vi "Motor controller.vi"   [LabVIEW 2012]
uses:
  Motors Values.vi
  BotStatus.vi
types:
  T1 = typedef "WPI_ServoDeviceRef.ctl" = cluster{"DeviceStatus":errorcluster, "Digital Module":T2, "PWM Channel":T3, "DeadBand":T4}
  T2 = typedef "FPGA_TypedefDigitalModule.ctl" = enum16{"Digital Module 1", "Digital Module 2"}
  T3 = typedef "FPGA_DIOPWMChannel.ctl" = enum8{"PWM 1", "PWM 2", "PWM 3", "PWM 4", "PWM 5", "PWM 6", "PWM 7", "PWM 8", "PWM 9", "PWM 10", "Invalid"}
  T4 = typedef "WPI_PWMDeadband.ctl" = cluster{"Name":string, "maxPositivePwm":i32, "minPositivePwm":i32, "centerPwm":i32, "maxNegativePwm":i32, "minNegativePwm":i32, "angularRange":u16}
  T5 = typedef "WPI_MotorControlDeviceRef.ctl" = cluster{"DeviceStatus":errorcluster, "Type":enum16{"PWM", "CAN"}, "PWM":cluster{"Digital Module":T2, "PWM Channel":T3, "DeadBand":T4}, "CAN":cluster{"Device Number":u8, "Control Mode":T6, "Semaphore":T7, "Max Vout":dbl}, "Invert":bool, "TransformRef":T8, "InvTransformRef":T8}
  T6 = typedef "WPI_CANJaguar_ControlMode.ctl" = enum8{"Percent VBus", "Current", "Speed", "Position", "Voltage"}
  T7 = typedef "Semaphore RefNum" = refnum<k1>
  T8 = typedef "WPI_PWMTransform_ConPane.ctl" = refnum<vi>
  T9 = typedef "WPI_RelayDevRef.ctl" = cluster{"DevStatus":errorcluster, "Relay Channel":T10, "Digital Module":T2, "Relay Direction":T11}
  T10 = typedef "FPGA_DIORelayChannel.ctl" = enum8{"Relay 1", "Relay 2", "Relay 3", "Relay 4", "Relay 5", "Relay 6", "Relay 7", "Relay 8", "Invalid"}
  T11 = typedef "WPI_RelayDirection.ctl" = enum16{"Both directions", "Forward only", "Reverse only"}
  T12 = typedef "WPI_RelayValue.ctl" = enum16{"Off", "On", "Forward", "Reverse"}
  T13 = typedef "WPI_DigitalInputDevRef.ctl" = cluster{"DevStatus":errorcluster, "DIO Channel":T14, "Digital Module":T2}
  T14 = typedef "FPGA_DIOChannel.ctl" = enum8{"DIO 1", "DIO 2", "DIO 3", "DIO 4", "DIO 5", "DIO 6", "DIO 7", "DIO 8", "DIO 9", "DIO 10", "DIO 11", "DIO 12", "DIO 13", "DIO 14", "Invalid"}
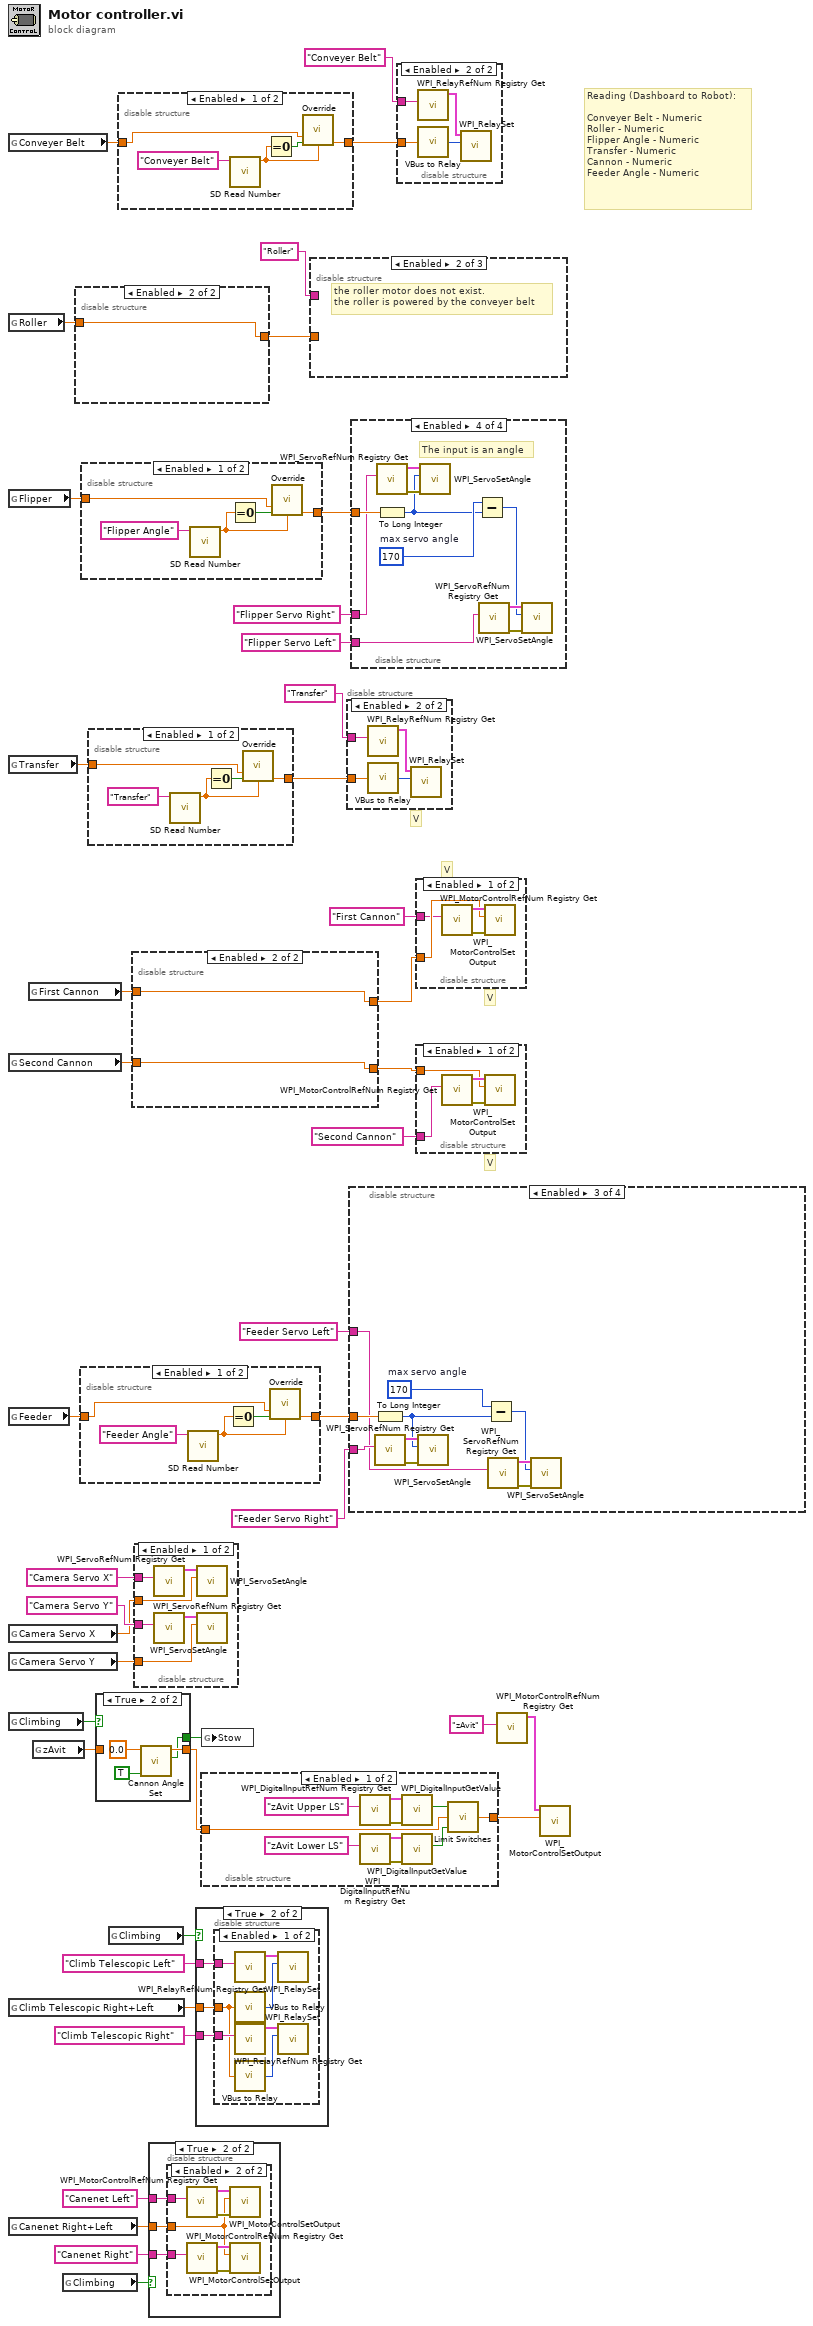
[diagram p0: block diagram]
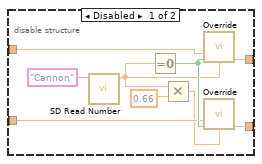
[diagram p4: hidden frame]
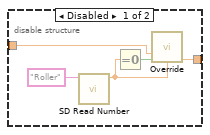
[diagram p7: hidden frame]
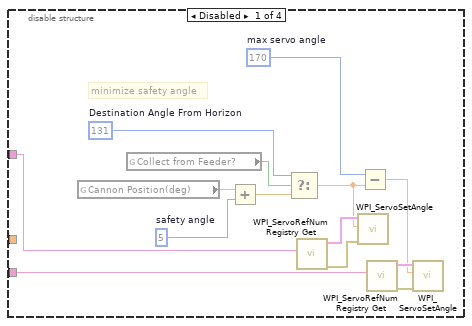
[diagram p10: hidden frame]
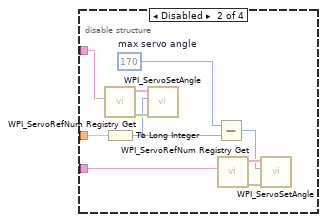
[diagram p11: hidden frame]
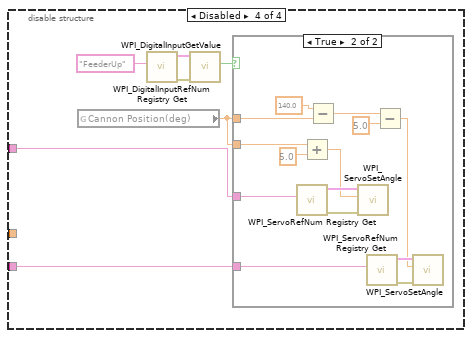
[diagram p12: hidden frame]
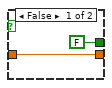
[diagram p14: hidden frame]
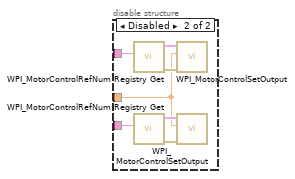
[diagram p18: hidden frame]
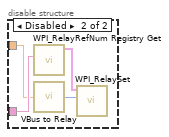
[diagram p19: hidden frame]
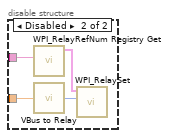
[diagram p20: hidden frame]
diagram:
  # "Reading (Dashboard to Robot):\n\nConveyer Belt - Numeric\nRoller - Numeric\nFlipper Angle - Numeric\nTransfer - Numeric\nCannon - Numeric\nFeeder Angle - Numeric"
  # "V"
  # "V"
  # "V"
  # "V"
  n1 = global read "Motors Values.vi" "Conveyer Belt"() -> (w15:dbl)
  n2 = global read "Motors Values.vi" "Roller"() -> (w14:dbl)
  n3 = global read "Motors Values.vi" "Flipper"() -> (w12:dbl)
  n4 = global read "Motors Values.vi" "Transfer"() -> (w10:dbl)
  n5 = global read "Motors Values.vi" "Second Cannon"() -> (w6:dbl)
  n6 = global read "Motors Values.vi" "Feeder"() -> (w3:dbl)
  n7 = global read "Motors Values.vi" "Camera Servo X"() -> (w18:dbl)
  n8 = global read "Motors Values.vi" "Camera Servo Y"() -> (w17:dbl)
  n9 = global read "BotStatus.vi" "Climbing"() -> (w26:bool)
  n10 = global read "Motors Values.vi" "Climb Telescopic Right+Left"() -> (w34:dbl)
  n11 = global read "Motors Values.vi" "Canenet Right+Left"() -> (w27:dbl)
  n12 = global read "Motors Values.vi" "First Cannon"() -> (w8:dbl)
  n13 = global read "Motors Values.vi" "zAvit"() -> (w25:dbl)
  n14 = global read "BotStatus.vi" "Climbing"() -> (w28:bool)
  n15 = disable-structure shown="Enabled" {
    disable-tunnel: w14 -> [w44 w48]
    disable-tunnel: [w43 w48] -> w13
    frame Disabled {
      n16 = call <vilib>:"SD Read Number.vi"("Name"="Roller") -> ("Numeric"=w46:dbl)  [unwired: 8 in, 2 out]
      n17 = Equal To 0?(x=w46) -> (x = 0?=w47:bool)
      n18 = call "Override.vi"("Regualer"=w44, "Override"=w47, "Overriden"=w46) -> ("Output"=w43:dbl)  [unwired: 12 in]
    }
    frame Enabled {
    }
  }
  n19 = disable-structure shown="Enabled" {
    disable-tunnel: [w50 w54] -> w4
    disable-tunnel: w3 -> [w49 w54]
    frame Enabled {
      n20 = call <vilib>:"SD Read Number.vi"("Name"="Feeder Angle") -> ("Numeric"=w53:dbl)  [unwired: 8 in, 2 out]
      n21 = Equal To 0?(x=w53) -> (x = 0?=w52:bool)
      n22 = call "Override.vi"("Regualer"=w49, "Override"=w52, "Overriden"=w53) -> ("Output"=w50:dbl)  [unwired: 12 in]
    }
    frame Disabled {
    }
  }
  n23 = disable-structure shown="Enabled" {
    disable-tunnel: w12 -> [w56 w60]
    disable-tunnel: [w55 w60] -> w11
    frame Enabled {
      n24 = call <vilib>:"SD Read Number.vi"("Name"="Flipper Angle") -> ("Numeric"=w58:dbl)  [unwired: 8 in, 2 out]
      n25 = Equal To 0?(x=w58) -> (x = 0?=w57:bool)
      n26 = call "Override.vi"("Regualer"=w56, "Override"=w57, "Overriden"=w58) -> ("Output"=w55:dbl)  [unwired: 12 in]
    }
    frame Disabled {
    }
  }
  n27 = disable-structure shown="Enabled" {
    disable-tunnel: w10 -> [w62 w66]
    disable-tunnel: [w61 w66] -> w9
    frame Enabled {
      n28 = call <vilib>:"SD Read Number.vi"("Name"="Transfer") -> ("Numeric"=w64:dbl)  [unwired: 8 in, 2 out]
      n29 = Equal To 0?(x=w64) -> (x = 0?=w63:bool)
      n30 = call "Override.vi"("Regualer"=w62, "Override"=w63, "Overriden"=w64) -> ("Output"=w61:dbl)  [unwired: 12 in]
    }
    frame Disabled {
    }
  }
  n31 = case shown="True" w26 {
    tunnel: [w68 w70] -> w2
    tunnel: w25 -> [w68 _]
    tunnel: [FALSE ("On Target") w69] -> w21
    frame False {
    }
    frame True {
      n32 = call "Cannon Angle Set.vi"("set angle 0 to be min angle"=TRUE, "Angle Set Point"=0.0) -> ("On Target"=w69:bool, "zAvit Vbus Out"=w70:dbl)  [unwired: 8 in]
    }
  }
  n33 = global read "BotStatus.vi" "Climbing"() -> (w33:bool)
  n34 = disable-structure shown="Enabled" {
    disable-tunnel: [w77 w78] -> w16
    disable-tunnel: w15 -> [w74 w78]
    frame Enabled {
      n35 = call <vilib>:"SD Read Number.vi"("Name"="Conveyer Belt") -> ("Numeric"=w75:dbl)  [unwired: 8 in, 2 out]
      n36 = Equal To 0?(x=w75) -> (x = 0?=w73:bool)
      n37 = call "Override.vi"("Regualer"=w74, "Override"=w73, "Overriden"=w75) -> ("Output"=w77:dbl)  [unwired: 12 in]
    }
    frame Disabled {
    }
  }
  n38 = disable-structure shown="Enabled" {
    disable-tunnel: w8 -> [w86 w89]
    disable-tunnel: [w85 w89] -> w7
    disable-tunnel: w6 -> [w83 w88]
    disable-tunnel: [w79 w88] -> w5
    frame Disabled {
      n39 = call <vilib>:"SD Read Number.vi"("Name"="Cannon") -> ("Numeric"=w82:dbl)  [unwired: 8 in, 2 out]
      n40 = Equal To 0?(x=w82) -> (x = 0?=w84:bool)
      n41 = Multiply(x=w82, y=0.66) -> (x*y=w81:dbl)
      n42 = call "Override.vi"("Regualer"=w86, "Override"=w84, "Overriden"=w82) -> ("Output"=w85:dbl)  [unwired: 12 in]
      n43 = call "Override.vi"("Regualer"=w83, "Override"=w84, "Overriden"=w81) -> ("Output"=w79:dbl)  [unwired: 12 in]
    }
    frame Enabled {
    }
  }
  n44 = disable-structure shown="Enabled" {
    disable-tunnel: "Camera Servo X" ("refnum name") -> [w94 _]
    disable-tunnel: "Camera Servo Y" ("refnum name") -> [w93 _]
    disable-tunnel: w18 -> [w91 _]
    disable-tunnel: w17 -> [w90 _]
    frame Enabled {
      n45 = call <vilib>:"WPI_ServoRefNum Registry Get.vi"("refnum name"=w94) -> ("ServoDeviceRef"=w95:T1)  [unwired: 9 in, 1 out]
      n46 = call <vilib>:"WPI_ServoRefNum Registry Get.vi"("refnum name"=w93) -> ("ServoDeviceRef"=w92:T1)  [unwired: 9 in, 1 out]
      n47 = call <vilib>:"WPI_ServoSetAngle.vi"("Angle"=w91, "ServoDeviceRef"=w95) -> ()  [unwired: 8 in, 2 out]
      n48 = call <vilib>:"WPI_ServoSetAngle.vi"("Angle"=w90, "ServoDeviceRef"=w92) -> ()  [unwired: 8 in, 2 out]
    }
    frame Disabled {
    }
  }
  n49 = case shown="True" w28 {
    tunnel: w27 -> [_ w98]
    tunnel: "Canenet Right" ("refnum name") -> [_ w97]
    tunnel: "Canenet Left" ("refnum name") -> [_ w96]
    frame False {
    }
    frame True {
      n50 = disable-structure shown="Enabled" {
        disable-tunnel: w98 -> [_ w99]
        disable-tunnel: w97 -> [_ w101]
        disable-tunnel: w96 -> [_ w100]
        frame Disabled {
        }
        frame Enabled {
          n51 = call <vilib>:"WPI_MotorControlRefNum Registry Get.vi"("refnum name"=w100) -> ("error out"=w102:errorcluster, "MotorControlDevRef"=w103:T5)  [unwired: 9 in]
          n52 = call <vilib>:"WPI_MotorControlRefNum Registry Get.vi"("refnum name"=w101) -> ("error out"=w105:errorcluster, "MotorControlDevRef"=w104:T5)  [unwired: 9 in]
          n53 = call <vilib>:"WPI_MotorControlSetOutput.vi"("error in (no error)"=w102, "Output"=w99, "MotorControlDevRef"=w103) -> ()  [unwired: 6 in, 3 out]
          n54 = call <vilib>:"WPI_MotorControlSetOutput.vi"("error in (no error)"=w105, "Output"=w99, "MotorControlDevRef"=w104) -> ()  [unwired: 6 in, 3 out]
        }
      }
    }
  }
  n55 = case shown="True" w33 {
    tunnel: w34 -> [_ w108]
    tunnel: "Climb Telescopic Right" ("refnum name") -> [_ w107]
    tunnel: "Climb Telescopic Left" ("refnum name") -> [_ w106]
    frame False {
    }
    frame True {
      n56 = disable-structure shown="Enabled" {
        disable-tunnel: w108 -> [w110 w116]
        disable-tunnel: w107 -> [w111 w118]
        disable-tunnel: w106 -> [w112 w117]
        frame Enabled {
          n57 = call <vilib>:"WPI_RelayRefNum Registry Get.vi"("refnum name"=w112) -> ("RelayDevRef"=w114:T9)  [unwired: 9 in, 1 out]
          n58 = call "VBus to Relay.vi"("Motor VBus"=w110) -> ("RelayValue"=w113:T12)  [unwired: 3 in]
          n59 = call <vilib>:"WPI_RelayRefNum Registry Get.vi"("refnum name"=w111) -> ("RelayDevRef"=w109:T9)  [unwired: 9 in, 1 out]
          n60 = call "VBus to Relay.vi"("Motor VBus"=w110) -> ("RelayValue"=w115:T12)  [unwired: 3 in]
          n61 = call <vilib>:"WPI_RelaySet.vi"("RelayValue"=w113, "RelayDevRef"=w114) -> ()  [unwired: 8 in, 2 out]
          n62 = call <vilib>:"WPI_RelaySet.vi"("RelayValue"=w115, "RelayDevRef"=w109) -> ()  [unwired: 8 in, 2 out]
        }
        frame Disabled {
          n63 = call <vilib>:"WPI_MotorControlRefNum Registry Get.vi"("refnum name"=w117) -> ("error out"=w119:errorcluster, "MotorControlDevRef"=w120:T5)  [unwired: 9 in]
          n64 = call <vilib>:"WPI_MotorControlRefNum Registry Get.vi"("refnum name"=w118) -> ("error out"=w122:errorcluster, "MotorControlDevRef"=w121:T5)  [unwired: 9 in]
          n65 = call <vilib>:"WPI_MotorControlSetOutput.vi"("error in (no error)"=w119, "Output"=w116, "MotorControlDevRef"=w120) -> ()  [unwired: 6 in, 3 out]
          n66 = call <vilib>:"WPI_MotorControlSetOutput.vi"("error in (no error)"=w122, "Output"=w116, "MotorControlDevRef"=w121) -> ()  [unwired: 6 in, 3 out]
        }
      }
    }
  }
  n67 = global write "BotStatus.vi" "Stow"(w21) -> ()
  n68 = disable-structure shown="Enabled" {
    disable-tunnel: w2 -> [w132 w133]
    disable-tunnel: [w131 w133] -> w1
    frame Enabled {
      n69 = call <vilib>:"WPI_DigitalInputRefNum Registry Get.vi"("refnum name"="zAvit Upper LS") -> ("error out"=w130:errorcluster, "DigitalInputDevRef"=w129:T13)  [unwired: 9 in]
      n70 = call <vilib>:"WPI_DigitalInputRefNum Registry Get.vi"("refnum name"="zAvit Lower LS") -> ("error out"=w128:errorcluster, "DigitalInputDevRef"=w127:T13)  [unwired: 9 in]
      n71 = call <vilib>:"WPI_DigitalInputGetValue.vi"("error in (no error)"=w130, "DigitalInputDevRef"=w129) -> ("Value"=w124:bool)  [unwired: 7 in, 2 out]
      n72 = call <vilib>:"WPI_DigitalInputGetValue.vi"("error in (no error)"=w128, "DigitalInputDevRef"=w127) -> ("Value"=w123:bool)  [unwired: 7 in, 2 out]
      n73 = call "Limit Switches.vi"("Backward Limit Switch"=w123, "VBus in"=w132, "Forward Limit Switch"=w124) -> ("VBus out"=w131:dbl)
    }
    frame Disabled {
    }
  }
  n74 = disable-structure shown="Enabled" {
    disable-tunnel: w13 -> [w135 _ w138]
    disable-tunnel: "Roller" ("refnum name") -> [w134 _ w140]
    frame Disabled {
      n75 = call <vilib>:"WPI_MotorControlRefNum Registry Get.vi"("refnum name"=w134) -> ("error out"=w137:errorcluster, "MotorControlDevRef"=w136:T5)  [unwired: 9 in]
      n76 = call <vilib>:"WPI_MotorControlSetOutput.vi"("error in (no error)"=w137, "Output"=w135, "MotorControlDevRef"=w136) -> ()  [unwired: 6 in, 3 out]
    }
    frame Enabled {
      # "the roller motor does not exist.\nthe roller is powered by the conveyer belt"
    }
    frame Disabled {
      n77 = call <vilib>:"WPI_RelayRefNum Registry Get.vi"("refnum name"=w140) -> ("RelayDevRef"=w139:T9)  [unwired: 9 in, 1 out]
      n78 = call "VBus to Relay.vi"("Motor VBus"=w138) -> ("RelayValue"=w141:T12)  [unwired: 3 in]
      n79 = call <vilib>:"WPI_RelaySet.vi"("RelayValue"=w141, "RelayDevRef"=w139) -> ()  [unwired: 8 in, 2 out]
    }
  }
  n80 = disable-structure shown="Enabled" {
    disable-tunnel: w9 -> [w143 w146]
    disable-tunnel: "Transfer" ("refnum name") -> [w142 w148]
    frame Disabled {
      n81 = call <vilib>:"WPI_MotorControlRefNum Registry Get.vi"("refnum name"=w142) -> ("error out"=w145:errorcluster, "MotorControlDevRef"=w144:T5)  [unwired: 9 in]
      n82 = call <vilib>:"WPI_MotorControlSetOutput.vi"("error in (no error)"=w145, "Output"=w143, "MotorControlDevRef"=w144) -> ()  [unwired: 6 in, 3 out]
    }
    frame Enabled {
      n83 = call <vilib>:"WPI_RelayRefNum Registry Get.vi"("refnum name"=w148) -> ("RelayDevRef"=w147:T9)  [unwired: 9 in, 1 out]
      n84 = call "VBus to Relay.vi"("Motor VBus"=w146) -> ("RelayValue"=w149:T12)  [unwired: 3 in]
      n85 = call <vilib>:"WPI_RelaySet.vi"("RelayValue"=w149, "RelayDevRef"=w147) -> ()  [unwired: 8 in, 2 out]
    }
  }
  n86 = disable-structure shown="Enabled" {
    disable-tunnel: "Feeder Servo Left" ("refnum name") -> [w160 w165 w174 w186]
    disable-tunnel: "Feeder Servo Right" ("refnum name") -> [w157 w164 w175 w185]
    disable-tunnel: w4 -> [_ w167 w177 _]
    frame Disabled {
      w152 = 131  # Destination Angle From Horizon
      w156 = 170  # max servo angle
      w161 = 5  # safety angle
      # "minimize safety angle"
      n87 = global read "BotStatus.vi" "Cannon Position(deg)"() -> (w150:dbl)
      n88 = global read "BotStatus.vi" "Collect from Feeder?"() -> (w151:bool)
      n89 = Add(x=w150, y=w161) -> (x+y=w153:dbl)
      n90 = Select(t=w152, s=w151, f=w153) -> (s? t:f=w154:dbl)
      n91 = call <vilib>:"WPI_ServoRefNum Registry Get.vi"("refnum name"=w160) -> ("error out"=w162:errorcluster, "ServoDeviceRef"=w163:T1)  [unwired: 9 in]
      n92 = call <vilib>:"WPI_ServoSetAngle.vi"("error in (no error)"=w162, "Angle"=w154, "ServoDeviceRef"=w163) -> ()  [unwired: 7 in, 2 out]
      n93 = Subtract(x=w156, y=w154) -> (x-y=w155:dbl)
      n94 = call <vilib>:"WPI_ServoRefNum Registry Get.vi"("refnum name"=w157) -> ("error out"=w158:errorcluster, "ServoDeviceRef"=w159:T1)  [unwired: 9 in]
      n95 = call <vilib>:"WPI_ServoSetAngle.vi"("error in (no error)"=w158, "Angle"=w155, "ServoDeviceRef"=w159) -> ()  [unwired: 7 in, 2 out]
    }
    frame Disabled {
      w169 = 170  # max servo angle
      n96 = call <vilib>:"WPI_ServoRefNum Registry Get.vi"("refnum name"=w165) -> ("error out"=w172:errorcluster, "ServoDeviceRef"=w173:T1)  [unwired: 9 in]
      n97 = To Long Integer(number=w167) -> (32bit integer=w166:i32)
      n98 = call <vilib>:"WPI_ServoSetAngle.vi"("error in (no error)"=w172, "Angle"=w166, "ServoDeviceRef"=w173) -> ()  [unwired: 7 in, 2 out]
      n99 = Subtract(x=w169, y=w166) -> (x-y=w168:i32)
      n100 = call <vilib>:"WPI_ServoRefNum Registry Get.vi"("refnum name"=w164) -> ("error out"=w170:errorcluster, "ServoDeviceRef"=w171:T1)  [unwired: 9 in]
      n101 = call <vilib>:"WPI_ServoSetAngle.vi"("error in (no error)"=w170, "Angle"=w168, "ServoDeviceRef"=w171) -> ()  [unwired: 7 in, 2 out]
    }
    frame Enabled {
      w179 = 170  # max servo angle
      n102 = To Long Integer(number=w177) -> (32bit integer=w176:i32)
      n103 = call <vilib>:"WPI_ServoRefNum Registry Get.vi"("refnum name"=w175) -> ("error out"=w182:errorcluster, "ServoDeviceRef"=w183:T1)  [unwired: 9 in]
      n104 = call <vilib>:"WPI_ServoSetAngle.vi"("error in (no error)"=w182, "Angle"=w176, "ServoDeviceRef"=w183) -> ()  [unwired: 7 in, 2 out]
      n105 = Subtract(x=w179, y=w176) -> (x-y=w178:i32)
      n106 = call <vilib>:"WPI_ServoRefNum Registry Get.vi"("refnum name"=w174) -> ("error out"=w180:errorcluster, "ServoDeviceRef"=w181:T1)  [unwired: 9 in]
      n107 = call <vilib>:"WPI_ServoSetAngle.vi"("error in (no error)"=w180, "Angle"=w178, "ServoDeviceRef"=w181) -> ()  [unwired: 7 in, 2 out]
    }
    frame Disabled {
      n108 = global read "BotStatus.vi" "Cannon Position(deg)"() -> (w184:dbl)
      n109 = call <vilib>:"WPI_DigitalInputRefNum Registry Get.vi"("refnum name"="FeederUp") -> ("error out"=w188:errorcluster, "DigitalInputDevRef"=w187:T13)  [unwired: 9 in]
      n110 = call <vilib>:"WPI_DigitalInputGetValue.vi"("error in (no error)"=w188, "DigitalInputDevRef"=w187) -> ("Value"=w190:bool)  [unwired: 7 in, 2 out]
      n111 = case shown="True" w190 {
        tunnel: w186 -> [_ w202]
        tunnel: w184 -> [_ w201]
        tunnel: w185 -> [_ w193]
        tunnel: w184 -> [_ w192]
        frame False {
        }
        frame True {
          n112 = call <vilib>:"WPI_ServoRefNum Registry Get.vi"("refnum name"=w202) -> ("error out"=w203:errorcluster, "ServoDeviceRef"=w204:T1)  [unwired: 9 in]
          n113 = Add(x=w201, y=5.0) -> (x+y=w199:dbl)
          n114 = Subtract(x=140.0, y=w192) -> (x-y=w197:dbl)
          n115 = call <vilib>:"WPI_ServoSetAngle.vi"("error in (no error)"=w203, "Angle"=w199, "ServoDeviceRef"=w204) -> ()  [unwired: 7 in, 2 out]
          n116 = call <vilib>:"WPI_ServoRefNum Registry Get.vi"("refnum name"=w193) -> ("error out"=w194:errorcluster, "ServoDeviceRef"=w195:T1)  [unwired: 9 in]
          n117 = Subtract(x=w197, y=5.0) -> (x-y=w191:dbl)
          n118 = call <vilib>:"WPI_ServoSetAngle.vi"("error in (no error)"=w194, "Angle"=w191, "ServoDeviceRef"=w195) -> ()  [unwired: 7 in, 2 out]
        }
      }
    }
  }
  n119 = disable-structure shown="Enabled" {
    disable-tunnel: w11 -> [w206 w209 w219 w230]
    disable-tunnel: "Flipper Servo Left" ("refnum name") -> [w205 w211 w222 w224]
    disable-tunnel: "Flipper Servo Right" ("refnum name") -> [_ _ w213 w223]
    frame Disabled {
      n120 = call <vilib>:"WPI_MotorControlRefNum Registry Get.vi"("refnum name"=w205) -> ("error out"=w208:errorcluster, "MotorControlDevRef"=w207:T5)  [unwired: 9 in]
      n121 = call <vilib>:"WPI_MotorControlSetOutput.vi"("error in (no error)"=w208, "Output"=w206, "MotorControlDevRef"=w207) -> ()  [unwired: 6 in, 3 out]
    }
    frame Disabled {
      n122 = call <vilib>:"WPI_RelayRefNum Registry Get.vi"("refnum name"=w211) -> ("RelayDevRef"=w210:T9)  [unwired: 9 in, 1 out]
      n123 = call "VBus to Relay.vi"("Motor VBus"=w209) -> ("RelayValue"=w212:T12)  [unwired: 3 in]
      n124 = call <vilib>:"WPI_RelaySet.vi"("RelayValue"=w212, "RelayDevRef"=w210) -> ()  [unwired: 8 in, 2 out]
    }
    frame Disabled {
      w216 = 170  # max servo angle
      # "The input is an angle"
      n125 = To Long Integer(number=w219) -> (32bit integer=w215:i32)
      n126 = call <vilib>:"WPI_ServoRefNum Registry Get.vi"("refnum name"=w222) -> ("error out"=w220:errorcluster, "ServoDeviceRef"=w221:T1)  [unwired: 9 in]
      n127 = call <vilib>:"WPI_ServoSetAngle.vi"("error in (no error)"=w220, "Angle"=w215, "ServoDeviceRef"=w221) -> ()  [unwired: 7 in, 2 out]
      n128 = Subtract(x=w216, y=w215) -> (x-y=w214:i32)
      n129 = call <vilib>:"WPI_ServoRefNum Registry Get.vi"("refnum name"=w213) -> ("error out"=w218:errorcluster, "ServoDeviceRef"=w217:T1)  [unwired: 9 in]
      n130 = call <vilib>:"WPI_ServoSetAngle.vi"("error in (no error)"=w218, "Angle"=w214, "ServoDeviceRef"=w217) -> ()  [unwired: 7 in, 2 out]
    }
    frame Enabled {
      w227 = 170  # max servo angle
      # "The input is an angle"
      n131 = call <vilib>:"WPI_ServoRefNum Registry Get.vi"("refnum name"=w223) -> ("error out"=w231:errorcluster, "ServoDeviceRef"=w232:T1)  [unwired: 9 in]
      n132 = To Long Integer(number=w230) -> (32bit integer=w226:i32)
      n133 = call <vilib>:"WPI_ServoSetAngle.vi"("error in (no error)"=w231, "Angle"=w226, "ServoDeviceRef"=w232) -> ()  [unwired: 7 in, 2 out]
      n134 = Subtract(x=w227, y=w226) -> (x-y=w225:i32)
      n135 = call <vilib>:"WPI_ServoRefNum Registry Get.vi"("refnum name"=w224) -> ("error out"=w229:errorcluster, "ServoDeviceRef"=w228:T1)  [unwired: 9 in]
      n136 = call <vilib>:"WPI_ServoSetAngle.vi"("error in (no error)"=w229, "Angle"=w225, "ServoDeviceRef"=w228) -> ()  [unwired: 7 in, 2 out]
    }
  }
  n137 = disable-structure shown="Enabled" {
    disable-tunnel: w16 -> [w234 w237]
    disable-tunnel: "Conveyer Belt" ("refnum name") -> [w233 w239]
    frame Disabled {
      n138 = call <vilib>:"WPI_MotorControlRefNum Registry Get.vi"("refnum name"=w233) -> ("error out"=w236:errorcluster, "MotorControlDevRef"=w235:T5)  [unwired: 9 in]
      n139 = call <vilib>:"WPI_MotorControlSetOutput.vi"("error in (no error)"=w236, "Output"=w234, "MotorControlDevRef"=w235) -> ()  [unwired: 6 in, 3 out]
    }
    frame Enabled {
      n140 = call <vilib>:"WPI_RelayRefNum Registry Get.vi"("refnum name"=w239) -> ("RelayDevRef"=w238:T9)  [unwired: 9 in, 1 out]
      n141 = call "VBus to Relay.vi"("Motor VBus"=w237) -> ("RelayValue"=w240:T12)  [unwired: 3 in]
      n142 = call <vilib>:"WPI_RelaySet.vi"("RelayValue"=w240, "RelayDevRef"=w238) -> ()  [unwired: 8 in, 2 out]
    }
  }
  n143 = disable-structure shown="Enabled" {
    disable-tunnel: w7 -> [w242 w245]
    disable-tunnel: "First Cannon" ("refnum name") -> [w241 w247]
    frame Enabled {
      n144 = call <vilib>:"WPI_MotorControlRefNum Registry Get.vi"("refnum name"=w241) -> ("error out"=w244:errorcluster, "MotorControlDevRef"=w243:T5)  [unwired: 9 in]
      n145 = call <vilib>:"WPI_MotorControlSetOutput.vi"("error in (no error)"=w244, "Output"=w242, "MotorControlDevRef"=w243) -> ()  [unwired: 6 in, 3 out]
    }
    frame Disabled {
      n146 = call <vilib>:"WPI_RelayRefNum Registry Get.vi"("refnum name"=w247) -> ("RelayDevRef"=w246:T9)  [unwired: 9 in, 1 out]
      n147 = call "VBus to Relay.vi"("Motor VBus"=w245) -> ("RelayValue"=w248:T12)  [unwired: 3 in]
      n148 = call <vilib>:"WPI_RelaySet.vi"("RelayValue"=w248, "RelayDevRef"=w246) -> ()  [unwired: 8 in, 2 out]
    }
  }
  n149 = disable-structure shown="Enabled" {
    disable-tunnel: w5 -> [w250 w253]
    disable-tunnel: "Second Cannon" ("refnum name") -> [w249 w255]
    frame Enabled {
      n150 = call <vilib>:"WPI_MotorControlRefNum Registry Get.vi"("refnum name"=w249) -> ("error out"=w252:errorcluster, "MotorControlDevRef"=w251:T5)  [unwired: 9 in]
      n151 = call <vilib>:"WPI_MotorControlSetOutput.vi"("error in (no error)"=w252, "Output"=w250, "MotorControlDevRef"=w251) -> ()  [unwired: 6 in, 3 out]
    }
    frame Disabled {
      n152 = call <vilib>:"WPI_RelayRefNum Registry Get.vi"("refnum name"=w255) -> ("RelayDevRef"=w254:T9)  [unwired: 9 in, 1 out]
      n153 = call "VBus to Relay.vi"("Motor VBus"=w253) -> ("RelayValue"=w256:T12)  [unwired: 3 in]
      n154 = call <vilib>:"WPI_RelaySet.vi"("RelayValue"=w256, "RelayDevRef"=w254) -> ()  [unwired: 8 in, 2 out]
    }
  }
  n155 = call <vilib>:"WPI_MotorControlRefNum Registry Get.vi"("refnum name"="zAvit") -> ("MotorControlDevRef"=w23:T5)  [unwired: 9 in, 1 out]
  n156 = call <vilib>:"WPI_MotorControlSetOutput.vi"("Output"=w1, "MotorControlDevRef"=w23) -> ()  [unwired: 7 in, 3 out]
